vi "GetTriggerStatus.vi"() -> ()   [LabVIEW 2015, in "Tektronix AFG 3000 Series.lvlib"]
uses:
  Tektronix AFG 3000 Series.lvlib
panel:
  out "internal trigger rate":dbl
  out "External Trigger Slope (0: Positive)  2":u16(ring) items=["Positive", "Negative"]
  out "Trigger Source (3:Internal)":u16(ring)=3 items=["Internal"=3, "EXT"=1]
  out "after substring":string
  out "read buffer":string
  out "VISA resource name out":refnum<visa-resource-name>
  out "error out":errorcluster
  in  "error in (no error)":errorcluster
  in  "VISA resource name":refnum<visa-resource-name>
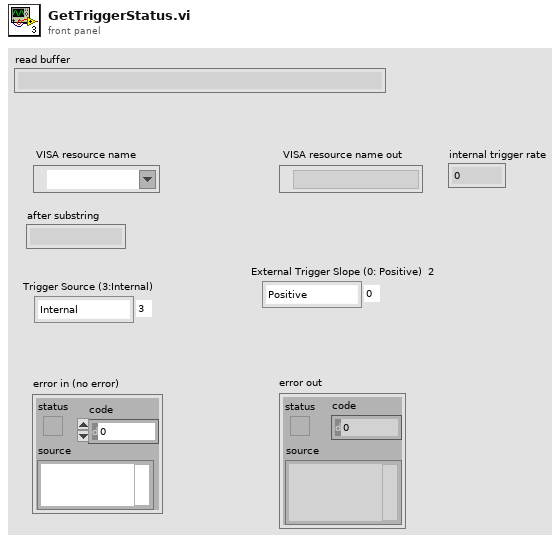
[diagram p1: front panel]
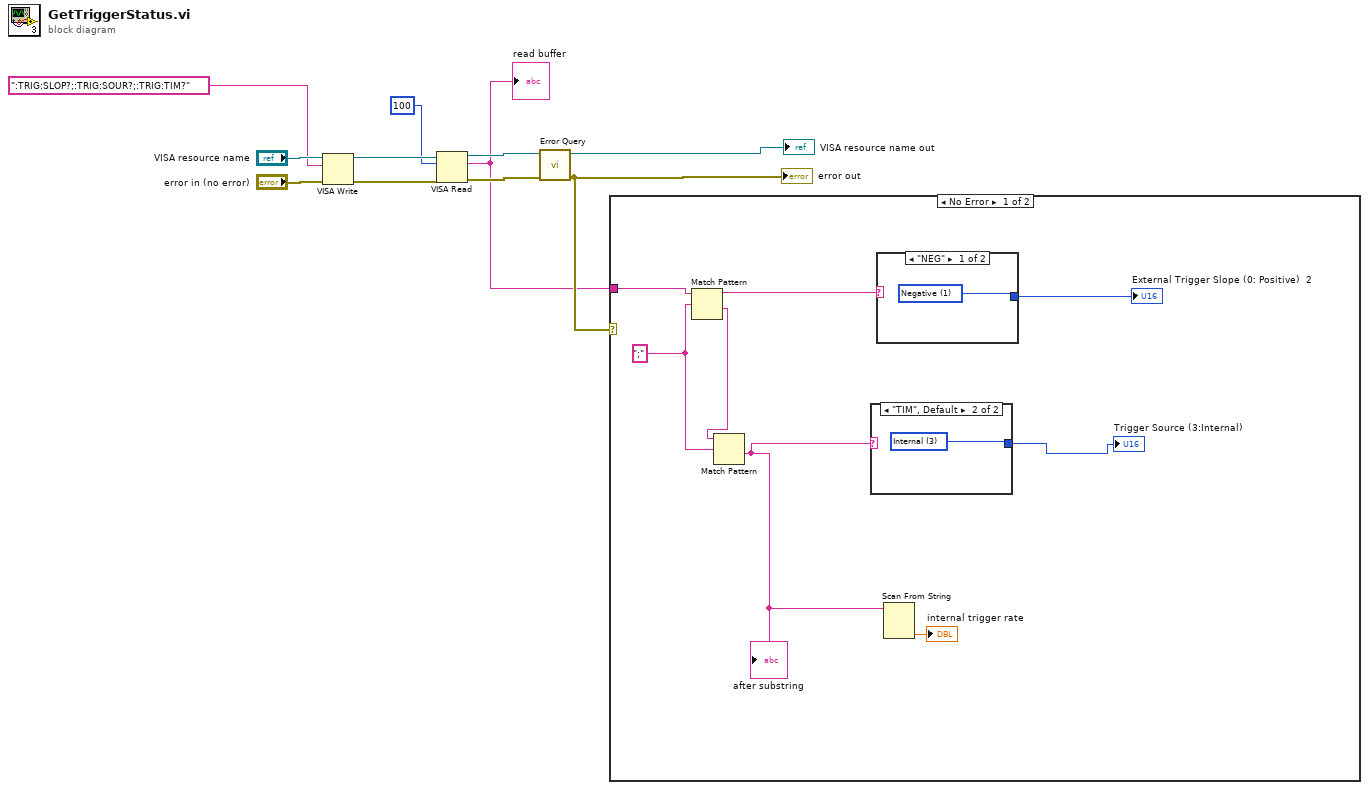
[diagram p0: block diagram]
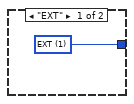
[diagram p2: hidden frame]
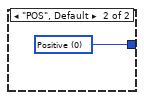
[diagram p3: hidden frame]
diagram:
  n1 = VISA Write(VISA resource name="VISA resource name", write buffer=":TRIG:SLOP?;:TRIG:SOUR?;:TRIG:TIM?", error in (no error)="error in (no error)") -> (VISA resource name out=w7:refnum<visa-resource-name>, error out=w4:errorcluster)  [unwired: 1 out]
  n2 = VISA Read(VISA resource name=w7, byte count=u32 100, error in (no error)=w4) -> (VISA resource name out=w6:refnum<visa-resource-name>, read buffer=w1:string, error out=w5:errorcluster)  [unwired: 1 out]
  "read buffer" <- w1
  n3 = call "Error Query.vi"("error in (no error)"=w5, "VISA resource name"=w6) -> ("error out"=w2:errorcluster, "VISA resource name out"=→"VISA resource name out":refnum<visa-resource-name>)  [unwired: 6 in, 2 out]
  "error out" <- w2
  n4 = case shown="No Error" w2 {
    tunnel: w1 -> [w19 _]
    frame No Error {
      w18 = ";" ("regular expression")
      n5 = Match Pattern(string=w19, regular expression=w18) -> (before substring=w16:string, after substring=w17:string)  [unwired: 1 in, 2 out]
      n6 = Match Pattern(string=w17, regular expression=w18) -> (after substring=w13:string)  [unwired: 1 in, 3 out]
      "after substring" <- w13
      n7 = case shown="\"TIM\", Default" w13 {
        tunnel: [w20 w21] -> w14
        frame "EXT" {
          w20 = u16 1 items=["Internal"=3, "EXT"=1] ("Trigger Source (3:Internal)")
        }
        frame "TIM", Default {
          w21 = u16 3 items=["Internal"=3, "EXT"=1] ("Trigger Source (3:Internal)")
        }
      }
      "Trigger Source (3:Internal)" <- w14
      n8 = case shown="\"NEG\"" w16 {
        tunnel: [w22 w23] -> w15
        frame "NEG" {
          w22 = u16 1 items=["Positive", "Negative"] ("External Trigger Slope (0: Positive)  2")
        }
        frame "POS", Default {
          w23 = u16 0 items=["Positive", "Negative"] ("External Trigger Slope (0: Positive)  2")
        }
      }
      "External Trigger Slope (0: Positive)  2" <- w15
      n9 = Scan From String(input string=w13) -> (output 1=→"internal trigger rate":dbl)  [unwired: 4 in, 3 out]
    }
    frame Error {
    }
  }
